vi "GetHistoramResultNames.vi"(7 "ProjectName":string="Prj", 10 "Analysis_Histogram_Parameter":T2={"Interval Range"={"Minimum"=0.0, "Maximum"=0.0}, "ROI Out"={"Global Rectangle"=[], "Contours"=[]}, "Number of Classes"=256} {"Interval Range"."Maximum" format="%.2f"; "Interval Range"."Minimum" format="%.2f"}, 11 "ROI_Name":string="ROI1") -> (3 "ResultNames":string[](array[string]))   [LabVIEW 2019]
uses:
  Controls/Histogram/Analysis_Histogram_Parameter.ctl
  Controls/Histogram/Analysis_Histogram_Result.ctl
panel:
  in  "Analysis_Histogram_Result":T1={"ROI"={"Global Rectangle"=[27, 55, 270, 147], "Contours"=[{"Contour Type"=0, "ROI Type"=3, "Points"=[27, 55, 270, 147]}]}, "Output value"=0.0, "Histogram Report"={"histogram"=[], "Minimal Value"=0.0, "Maximal Value"=0.0, "Starting Value"=0.0, "Interval Width"=0.0, "Mean Value"=0.0, "Standard  Variation"=0.0, "Area (pixels)"=0}} {"Histogram Report"."Standard  Variation" format="%.2f"; "Histogram Report"."Mean Value" format="%.2f"; "Histogram Report"."Interval Width" format="%.2f"; "Histogram Report"."Starting Value" format="%.2f"; "Histogram Report"."Maximal Value" format="%.2f"; "Histogram Report"."Minimal Value" format="%.2f"}
  out "error out":errorcluster
  in  "error in (no error)":errorcluster
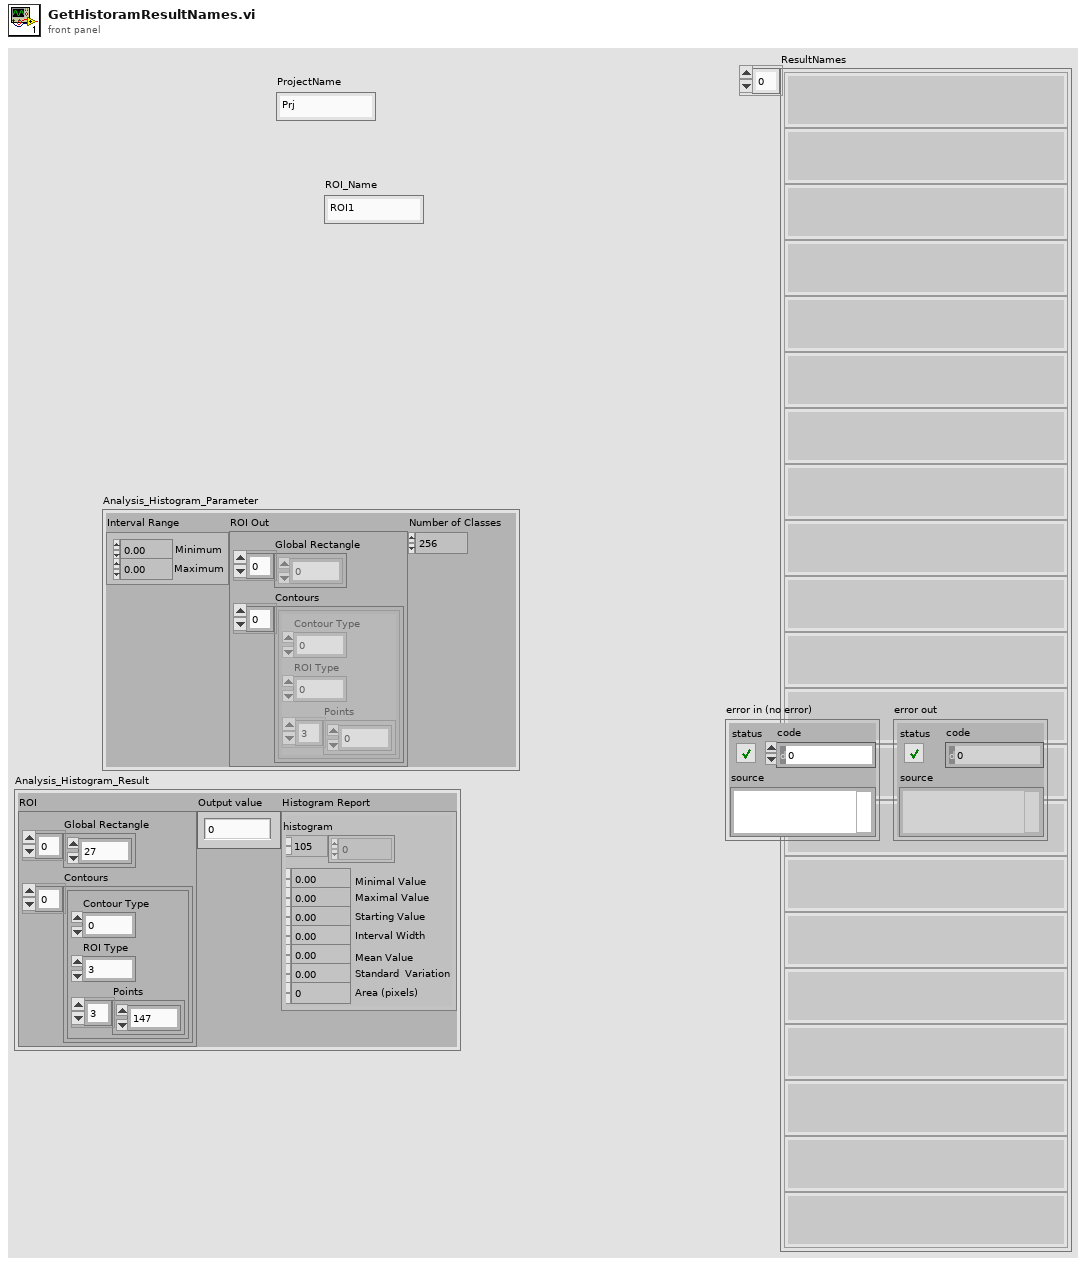
[diagram p1: front panel]
types:
  T1 = typedef "Analysis_Histogram_Result.ctl" = cluster{"ROI":cluster{"Global Rectangle":i32[], "Contours":cluster{"Contour Type":u32, "ROI Type":u32, "Points":i32[]}[]}, "Output value":dbl, "Histogram Report":cluster{"histogram":u32[], "Minimal Value":sgl, "Maximal Value":sgl, "Starting Value":sgl, "Interval Width":sgl, "Mean Value":sgl, "Standard  Variation":sgl, "Area (pixels)":i32}}
  T2 = typedef "Analysis_Histogram_Parameter.ctl" = cluster{"Interval Range":cluster{"Minimum":sgl, "Maximum":sgl}, "ROI Out":cluster{"Global Rectangle":i32[], "Contours":cluster{"Contour Type":u32, "ROI Type":u32, "Points":i32[]}[]}, "Number of Classes":i32}
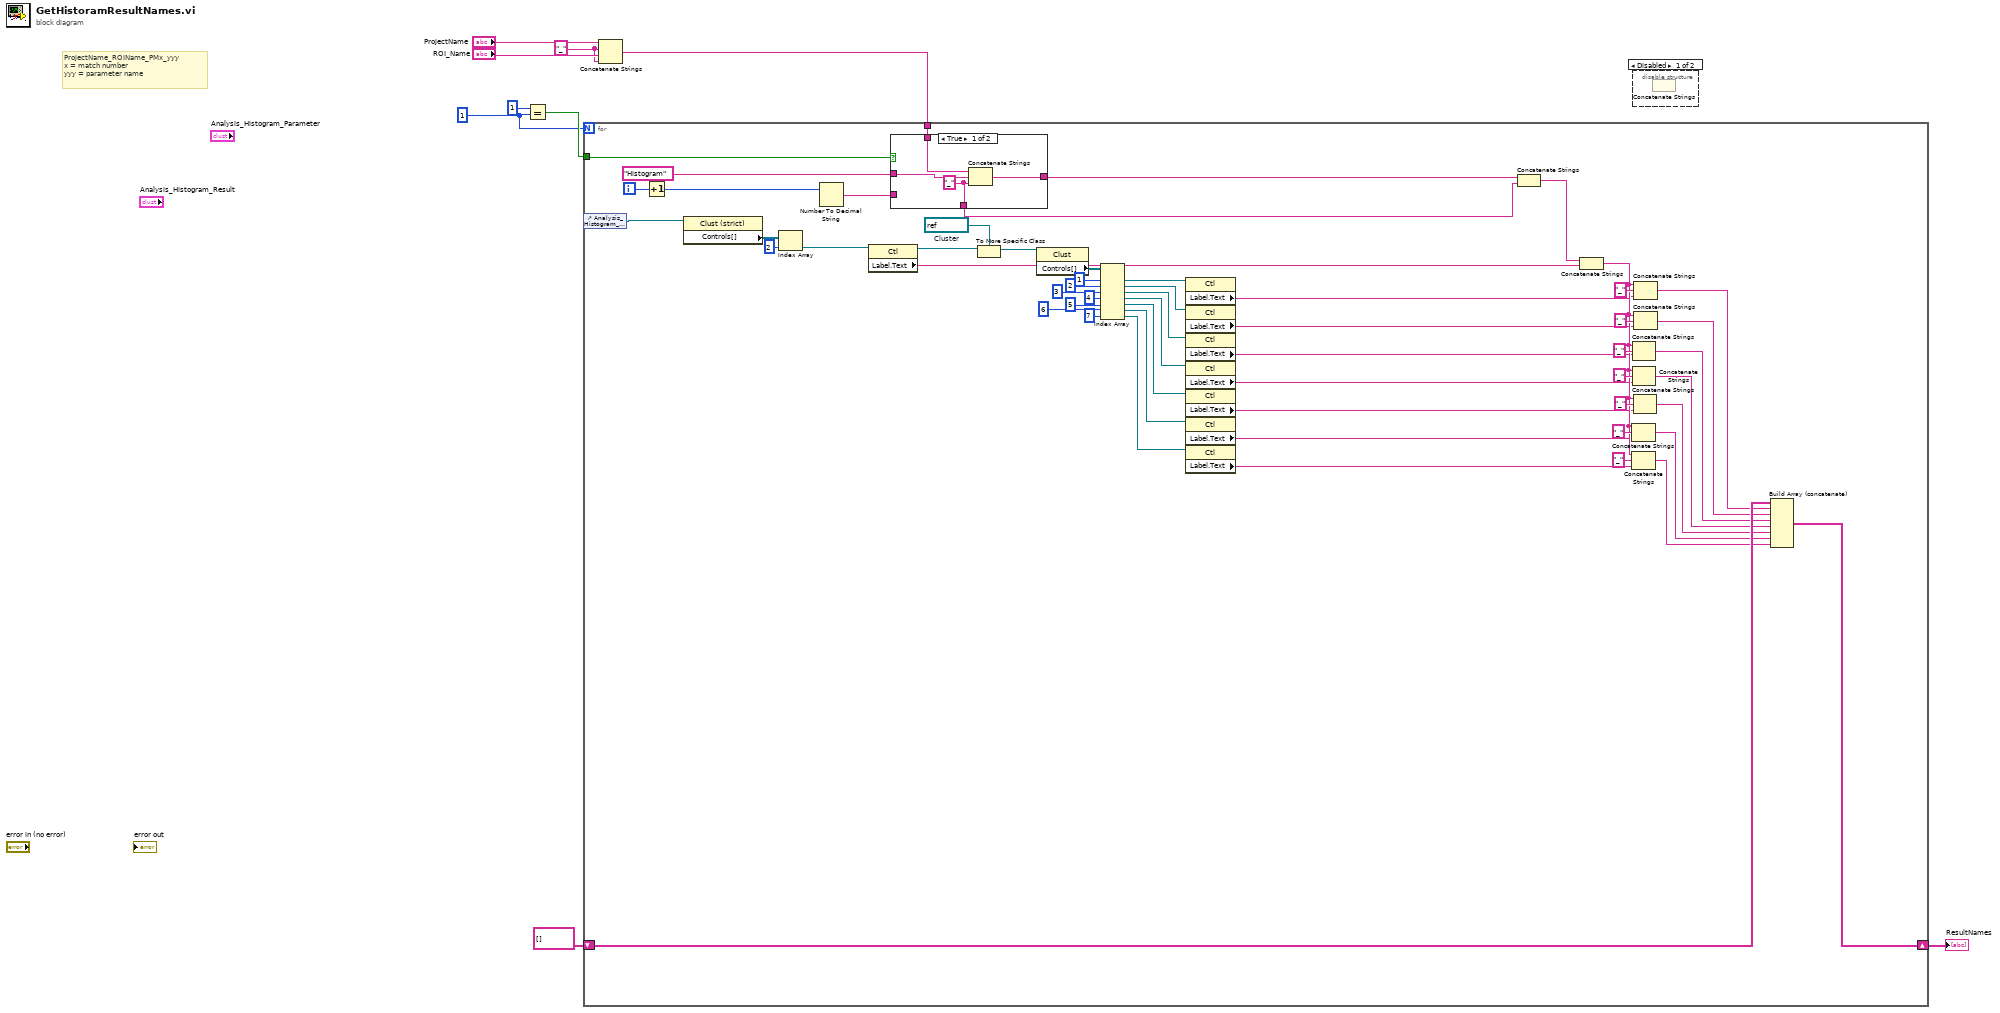
[diagram p0: block diagram]
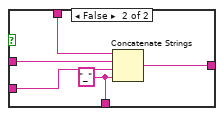
[diagram p3: hidden frame]
diagram:
  w1 = 1
  w7 = "_" ("string")
  # "ProjectName_ROIName_PMx_yyy\nx = match number\nyyy = parameter name"
  n1 = Equal?(x=1, y=w1) -> (x = y?=w3:bool)
  n2 = Concatenate Strings("ProjectName", w7, "ROI_Name", w7) -> (w6:string)
  n3 = for {
    N: w1 -> [_]
    tunnel: w6 -> [w63]
    shift-right: [w56] -> w4
    shift-left: string[] [] -> [w59]
    tunnel: w3 -> [w64]
    i -> [w60]
    w48 = refnum<vi> refnum  # Cluster
    n4 = control-ref of="Analysis_Histogram_Result"() -> (w51:refnum<vi>)
    n5 = Increment(x=w60) -> (x+1=w65:i32)
    n6 = property class="Clust (strict)"(reference=w51) -> ("Controls[]"=w58:refnum<vi>[])  [unwired: 1 in, 2 out]
    n7 = Index Array(array=w58, index=2) -> (element=w55:refnum<vi>)
    n8 = Number To Decimal String(number=w65) -> (decimal integer string=w62:string)  [unwired: 1 in]
    n9 = property class="Ctl"(reference=w55) -> (reference out=w49:refnum<vi>, "Label.Text"=w54:string)  [unwired: 1 in, 1 out]
    n10 = case shown="True" w64 {
      tunnel: w63 -> [w69 w74]
      tunnel: w62 -> [_ w72]
      tunnel: [w68 w73] -> w53
      tunnel: "Histogram" ("string") -> [w67 w71]
      tunnel: [w66 w70] -> w52
      frame True {
        w66 = "_" ("string")
        n11 = Concatenate Strings(w69, w67, w66) -> (w68:string)
      }
      frame False {
        w70 = "_" ("string")
        n12 = Concatenate Strings(w74, w71, w72, w70) -> (w73:string)
      }
    }
    n13 = To More Specific Class(target class=w48, reference=w49) -> (specific class reference=w47:refnum<vi>)  [unwired: 1 in, 1 out]
    n14 = property class="Clust"(reference=w47) -> ("Controls[]"=w46:refnum<vi>[])  [unwired: 1 in, 2 out]
    n15 = Index Array(array=w46, index #1=1 ("index"), index #2=2 ("index"), index #3=3 ("index"), index #4=4 ("index"), index #5=5 ("index"), index #6=6 ("index"), index #7=7 ("index")) -> (element #1=w45:refnum<vi>, element #2=w44:refnum<vi>, element #3=w43:refnum<vi>, element #4=w42:refnum<vi>, element #5=w41:refnum<vi>, element #6=w40:refnum<vi>, element #7=w39:refnum<vi>)
    n16 = property class="Ctl"(reference=w45) -> ("Label.Text"=w23:string)  [unwired: 1 in, 2 out]
    n17 = property class="Ctl"(reference=w44) -> ("Label.Text"=w22:string)  [unwired: 1 in, 2 out]
    n18 = property class="Ctl"(reference=w43) -> ("Label.Text"=w21:string)  [unwired: 1 in, 2 out]
    n19 = property class="Ctl"(reference=w42) -> ("Label.Text"=w20:string)  [unwired: 1 in, 2 out]
    n20 = property class="Ctl"(reference=w41) -> ("Label.Text"=w19:string)  [unwired: 1 in, 2 out]
    n21 = property class="Ctl"(reference=w40) -> ("Label.Text"=w18:string)  [unwired: 1 in, 2 out]
    n22 = property class="Ctl"(reference=w39) -> ("Label.Text"=w17:string)  [unwired: 1 in, 2 out]
    n23 = Concatenate Strings(w53, w52) -> (w50:string)
    n24 = Concatenate Strings(w50, w54) -> (w24:string)
    n25 = Concatenate Strings(w24, "_" ("string"), w18) -> (w11:string)
    n26 = Concatenate Strings(w24, "_" ("string"), w17) -> (w10:string)
    n27 = Concatenate Strings(w24, "_" ("string"), w21) -> (w14:string)
    n28 = Concatenate Strings(w24, "_" ("string"), w20) -> (w13:string)
    n29 = Concatenate Strings(w24, "_" ("string"), w19) -> (w12:string)
    n30 = Concatenate Strings(w24, "_" ("string"), w23) -> (w16:string)
    n31 = Concatenate Strings(w24, "_" ("string"), w22) -> (w15:string)
    n32 = Build Array (concatenate)(w59, w16, w15, w14, w13, w12, w11, w10) -> (w56:string[])
  }
  "ResultNames" <- w4
  n33 = disable-structure shown="Disabled" {
    frame Disabled {
      n34 = Concatenate Strings() -> ()  [unwired: 2 in, 1 out]
    }
    frame Enabled {
    }
  }
